vi "Structures 1.vi"() -> ()   [LabVIEW 2011]
panel:
  out "Carry":bool
  out "Sum":bool
  in  "C":bool
  in  "B":bool
  in  "A":bool
  in  "Boolean Control":bool
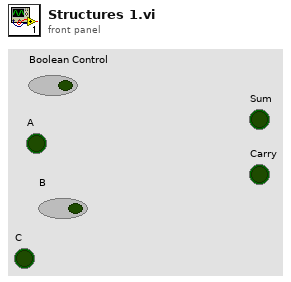
[diagram p1: front panel]
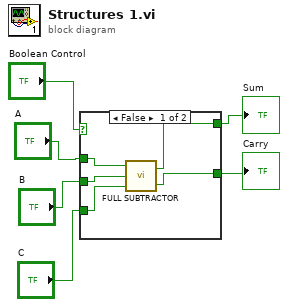
[diagram p0: block diagram]
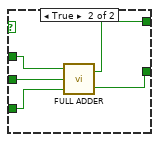
[diagram p2: hidden frame]
diagram:
  n1 = case shown="False" "Boolean Control" {
    tunnel: "A" -> [w11 w16]
    tunnel: "B" -> [w10 w15]
    tunnel: "C" -> [w9 w14]
    tunnel: [w8 w13] -> w2
    tunnel: [w7 w12] -> w1
    frame False {
      n2 = call "FULL SUBTRACTOR.vi"("C"=w9, "B"=w10, "A"=w11) -> ("BORROW"=w7:bool, "DIFF"=w8:bool)
    }
    frame True {
      n3 = call "FULL ADDER.vi"("C"=w14, "B"=w15, "A"=w16) -> ("CARRY"=w12:bool, "SUM"=w13:bool)
    }
  }
  "Sum" <- w2
  "Carry" <- w1
